vi "Superimpose Fiducial Indicator.vi"(6 "Marker Color":u32(colorbox)=16711680, 7 "size(pixels)":i32=20, 8 "error in":errorcluster, 9 "Clear Previous Overlay":bool=TRUE, 10 "Fiducial Image Coordinates":refnum<class "Vec3d Class.lvclass">, 11 "Image In":T1) -> (0 "error out":errorcluster, 3 "Image Out":T1)   [LabVIEW 2011]
uses:
  <vilib>/vision/Image Controls.llb/IMAQ Image.ctl
  Vec3d Class/Vec3d Class.lvclass
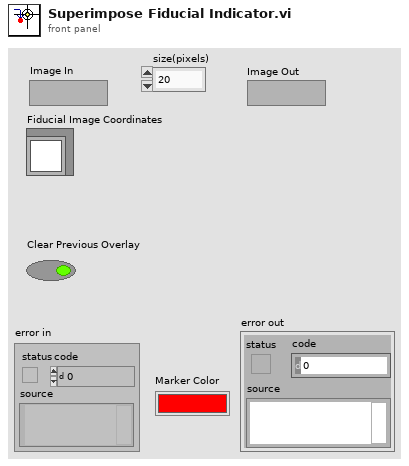
[diagram p1: front panel]
types:
  T1 = typedef "IMAQ Image.ctl" = refnum<image>
  T2 = cluster{"Left":i32, "Top":i32, "Right":i32, "Bottom":i32}
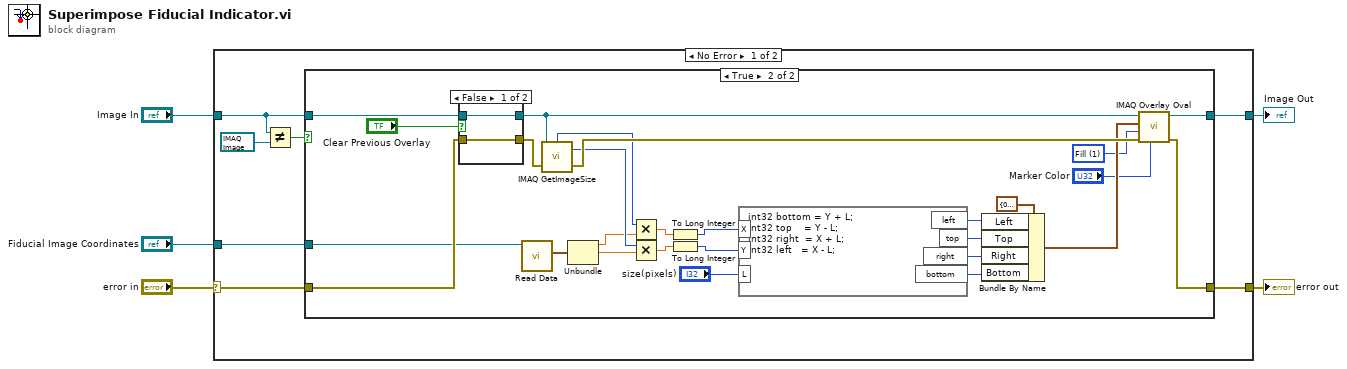
[diagram p0: block diagram]
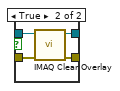
[diagram p3: hidden frame]
diagram:
  n1 = case shown="No Error" "error in" {
    selector: "error in" -> [w12 w49]
    tunnel: "Image In" -> [w7 w48]
    tunnel: [w9 w49] -> w3
    tunnel: "Fiducial Image Coordinates" -> [w11 _]
    tunnel: [w10 w48] -> w1
    frame No Error {
      n2 = Not Equal?(x=w7, y=T1 refnum ("Image In")) -> (x != y?=w6:bool)
      n3 = case shown="True" w6 {
        tunnel: w7 -> [w14 w41]
        tunnel: w12 -> [w13 w40]
        tunnel: w11 -> [_ w37]
        tunnel: [w14 w24] -> w10
        tunnel: [w13 w23] -> w9
        frame False {
        }
        frame True {
          w22 = u32 1 items=["Frame", "Fill"] ("Drawing Mode (Frame)")
          n4 = case shown="False" "Clear Previous Overlay" {
            tunnel: w41 -> [w43 w47]
            tunnel: w40 -> [w42 w46]
            tunnel: [w42 w45] -> w39
            tunnel: [w43 w44] -> w38
            frame False {
            }
            frame True {
              n5 = call "IMAQ Clear Overlay"("error in (no error)"=w46, "Image"=w47) -> ("error out"=w45:errorcluster, "Image Out"=w44:T1)  [unwired: 8 in]
            }
          }
          n6 = call-dynamic "Read Data.vi"("Vec3d Class in"=w37) -> ("Data"=w34:cluster{"X":dbl, "Y":dbl, "Z":dbl})  [unwired: 8 in, 2 out]
          n7 = call "IMAQ GetImageSize"("Image"=w38, "error in (no error)"=w39) -> ("Y Resolution"=w33:i32, "X Resolution"=w32:i32, "error out"=w36:errorcluster)  [unwired: 2 in]
          n8 = Unbundle(w34) -> ("X"=w20:dbl, "Y"=w21:dbl)  [unwired: 1 out]
          n9 = Multiply(x=w32, y=w20) -> (x*y=w19:dbl)
          n10 = Multiply(x=w33, y=w21) -> (x*y=w18:dbl)
          n11 = To Long Integer(number=w19) -> (32bit integer=w17:i32)
          n12 = To Long Integer(number=w18) -> (32bit integer=w16:i32)
          n13 = formula code="int32 bottom = Y + L;\nint32 top    = Y - L;\nint32 right  = X + L;\nint32 left   = X - L;"("X"=w17, "Y"=w16, "L"="size(pixels)") -> ("left"=w31:i32, "top"=w30:i32, "right"=w29:i32, "bottom"=w28:i32)
          n14 = Bundle By Name(cluster=T2 {"Left"=0, "Top"=0, "Right"=0, "Bottom"=0} ("Bounding Rectangle"), "Left"=w31, "Top"=w30, "Right"=w29, "Bottom"=w28) -> (w27:T2)
          n15 = call "IMAQ Overlay Oval"("Color"="Marker Color", "error in (no error)"=w36, "Drawing Mode (Frame)"=w22, "Bounding Rectangle"=w27, "Image"=w38) -> ("error out"=w23:errorcluster, "Image Out"=w24:T1)  [unwired: 5 in]
        }
      }
    }
    frame Error {
    }
  }
  "error out" <- w3
  "Image Out" <- w1
